vi "실습 2-6, Jog 제어.vi"() -> ()   [LabVIEW 2014]
uses:
  <vilib>/Motion/FlexMotion/CustomControls/CustomControls.llb/AxisOrVectorSpace To Configure.flx
  <vilib>/Motion/FlexMotion/FunctionsVIs/StartStopMotion.llb/Stop Motion (8 axes).flx
  <vilib>/Motion/FlexMotion/FunctionsVIs/StartStopMotion.llb/Start Motion (8 axes).flx
panel:
  in  "CW":bool
  in  "CCW":bool
  in  "정지":bool
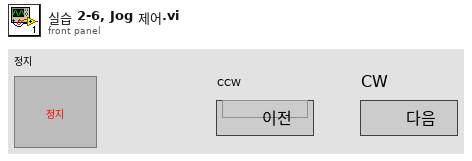
[diagram p1: front panel]
types:
  T1 = enum16{"Absolute Position", "Relative Position", "Velocity", "Relative to Cap Pos", "Modulus Position", "Absolute Contouring", "Relative Contouring"}
  T2 = typedef "AxisOrVectorSpace To Configure.flx" = u16
  T3 = typedef "Resource Out (Enum).flx" = u16
  T4 = typedef "Bd Id Out" = u8
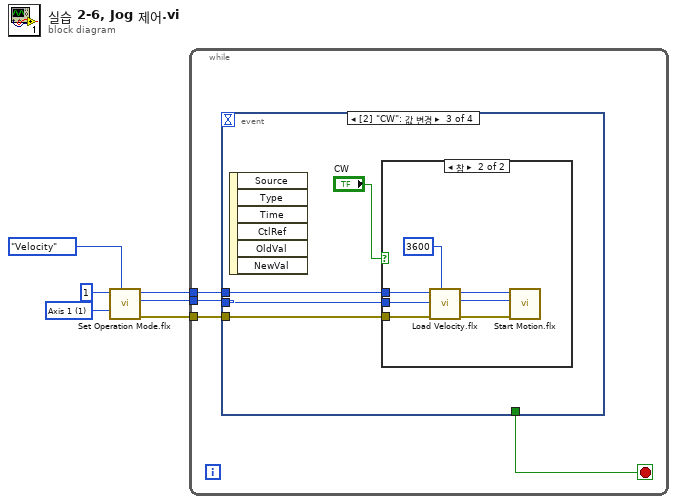
[diagram p0: block diagram]
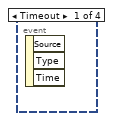
[diagram p2: hidden frame]
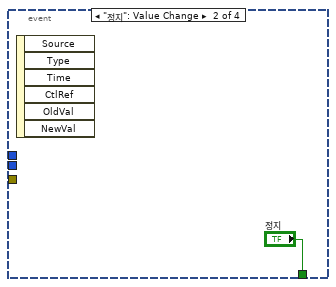
[diagram p3: hidden frame]
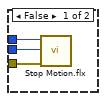
[diagram p4: hidden frame]
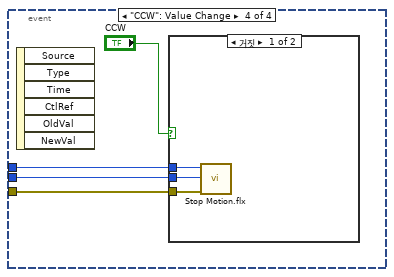
[diagram p5: hidden frame]
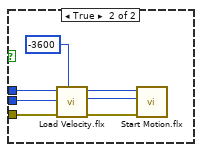
[diagram p6: hidden frame]
diagram:
  w5 = T2 1 items=["Axis 1"=1, "Axis 2"=2, "Axis 3"=3, "Axis 4"=4, "Axis 5"=5, "Axis 6"=6, "Axis 7"=7, "Axis 8"=8, "Vector Space 1"=17, "Vector Space 2"=18, "Vector Space 3"=19, "Vector Space 4"=20] ("Axis or Vector Space")
  n1 = call <vilib>:"Set Operation Mode.flx"("Position Mode (Absolute)"=T1."Velocity", "Axis or Vector Space"=w5, "Board ID"=u8 1) -> ("error out"=w1:errorcluster, "Resource Output"=w2:T3, "Bd ID Out"=w3:T4)  [unwired: 3 in]
  n2 = while {
    tunnel: w3 -> [w10]
    tunnel: w2 -> [w9]
    tunnel: w1 -> [w8]
    stop <- w7 stop-if-true
    n3 = event shown="[2] \"CW\": 값 변경" {
      selector: _ -> [_ _ _ _]
      dyn-events: _ -> [_ _ _ _]
      timeout: _ -> [_ _ _ _]
      tunnel: w10 -> [_ _ w14 w29]
      tunnel: w9 -> [_ _ w13 w28]
      tunnel: w8 -> [_ _ w12 w27]
      tunnel: [_ "정지" _ _] -> w7
      event Timeout {
        n4 = event-data() -> ()  [unwired: 1 in, 3 out]
      }
      event "정지": Value Change {
        n5 = event-data() -> ()  [unwired: 1 in, 6 out]
      }
      event "CW": Value Change {
        n6 = event-data() -> ()  [unwired: 1 in, 6 out]
        n7 = case shown="참" "CW" {
          tunnel: w14 -> [w17 w22]
          tunnel: w13 -> [w16 w21]
          tunnel: w12 -> [w18 w20]
          frame False {
            n8 = call-poly <vilib>:"Stop Motion.flx"("error in (no error)"=w18, "Axis or Vector Space"=w16, "Board ID"=w17) -> ()  [unwired: 4 in, 3 out]
          }
          frame True {
            n9 = call <vilib>:"Load Velocity.flx"("Velocity (10000)"=3600, "error in (no error)"=w20, "Axis or Vector Space"=w21, "Board ID"=w22) -> ("error out"=w23:errorcluster, "Resource Output"=w24:T3, "Bd ID Out"=w25:T4)  [unwired: 3 in]
            n10 = call-poly <vilib>:"Start Motion.flx"("error in (no error)"=w23, "Axis or Vector Space"=w24, "Board ID"=w25) -> ()  [unwired: 3 in, 3 out]
          }
        }
      }
      event "CCW": Value Change {
        n11 = event-data() -> ()  [unwired: 1 in, 6 out]
        n12 = case shown="거짓" "CCW" {
          tunnel: w29 -> [w31 w36]
          tunnel: w28 -> [w30 w35]
          tunnel: w27 -> [w32 w34]
          frame False {
            n13 = call-poly <vilib>:"Stop Motion.flx"("error in (no error)"=w32, "Axis or Vector Space"=w30, "Board ID"=w31) -> ()  [unwired: 4 in, 3 out]
          }
          frame True {
            n14 = call <vilib>:"Load Velocity.flx"("Velocity (10000)"=-3600, "error in (no error)"=w34, "Axis or Vector Space"=w35, "Board ID"=w36) -> ("error out"=w37:errorcluster, "Resource Output"=w38:T3, "Bd ID Out"=w39:T4)  [unwired: 3 in]
            n15 = call-poly <vilib>:"Start Motion.flx"("error in (no error)"=w37, "Axis or Vector Space"=w38, "Board ID"=w39) -> ()  [unwired: 3 in, 3 out]
          }
        }
      }
    }
  }
